vi "getRandomY.vi"(8 "error in (no error)":errorcluster, 11 "Flightweight Pattern Demo in":refnum<class "Flightweight Pattern Demo.lvclass">) -> (0 "error out":errorcluster, 2 "Y":i32, 3 "Flightweight Pattern Demo out":refnum<class "Flightweight Pattern Demo.lvclass">)   [LabVIEW 2016, in "Flightweight Pattern Demo.lvclass"]
uses:
  Flightweight Pattern Demo.lvclass
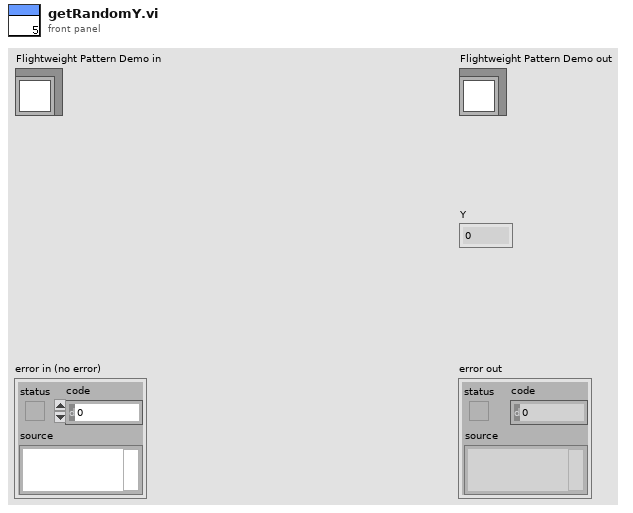
[diagram p1: front panel]
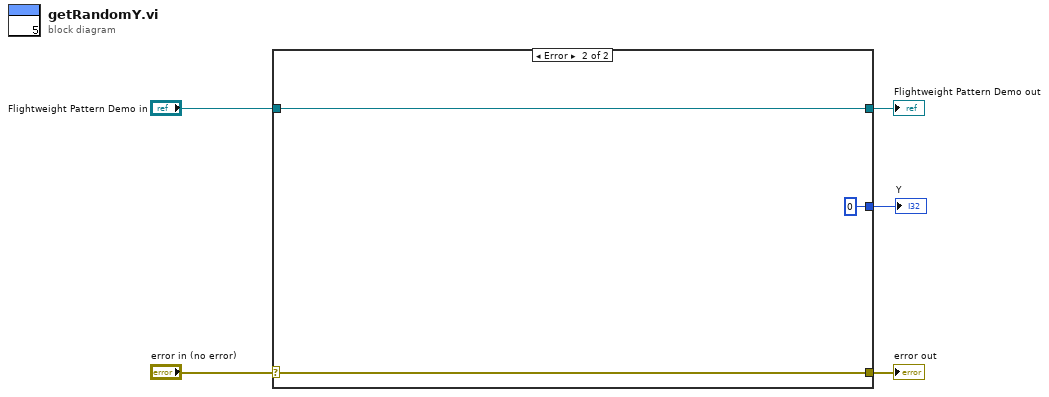
[diagram p0: block diagram]
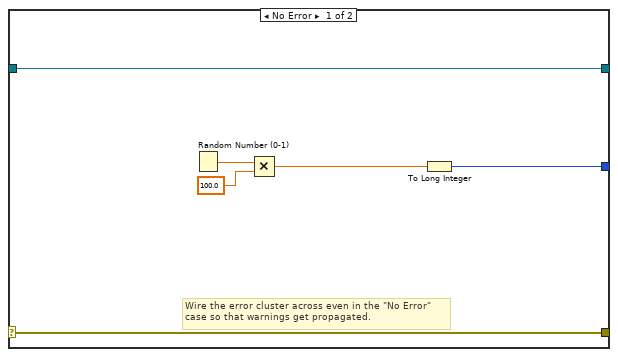
[diagram p2: hidden frame]
diagram:
  n1 = case shown="Error" "error in (no error)" {
    selector: "error in (no error)" -> [w10 w14]
    tunnel: [w10 w14] -> w4
    tunnel: [w11 w13] -> w2
    tunnel: "Flightweight Pattern Demo in" -> [w11 w13]
    tunnel: [w6 0] -> w1
    frame No Error {
      # "Wire the error cluster across even in the \"No Error\"\ncase so that warnings get propagated."
      n2 = Random Number (0-1)() -> (number: 0 to 1=w9:dbl)
      n3 = Multiply(x=w9, y=100.0) -> (x*y=w7:dbl)
      n4 = To Long Integer(number=w7) -> (32bit integer=w6:i32)
    }
    frame Error {
    }
  }
  "error out" <- w4
  "Flightweight Pattern Demo out" <- w2
  "Y" <- w1
